vi "EHL Undo Filter - Value Change MHLC.vi"(8 "error in (no error)":errorcluster, 11 "Message Log in":refnum<class "Message Log.lvclass">) -> (0 "error out":errorcluster, 3 "Message Log out":refnum<class "Message Log.lvclass">)   [LabVIEW 2017, in "Message Log.lvclass"]
doc: "Remove last applied filter"
uses:
  Message Log.lvclass
  Message Log.lvclass/Message Log.ctl
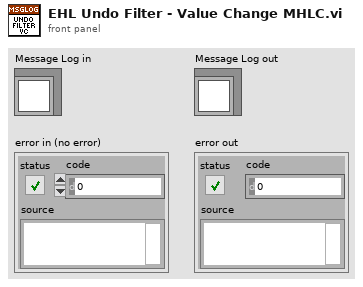
[diagram p1: front panel]
types:
  T1 = typedef "Message Log.lvclass/Message Log Filter Data.ctl" = cluster{"Element":string, "Column":T2, "Filter Type":T3}
  T2 = typedef "Message Log.lvclass/Message Log Columns.ctl" = enum16{"Count (sec)", "Time/Date", "Enque Worker", "Enque Case", "Deque Worker", "Deque Case", "Priority", "Message"}
  T3 = typedef "Message Log.lvclass/String Filter Type.ctl" = enum16{"string only", "match pattern"}
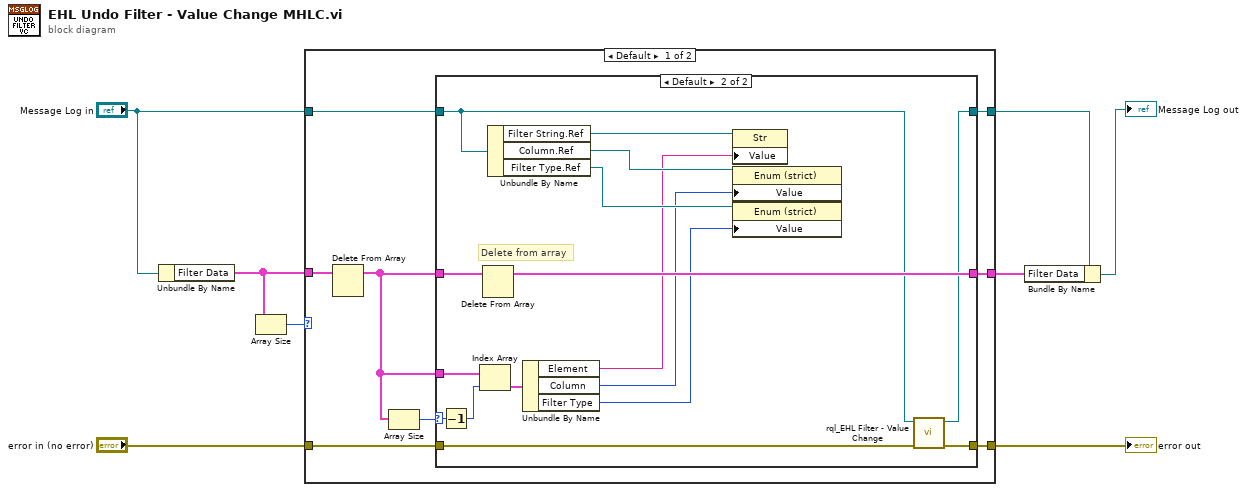
[diagram p0: block diagram]
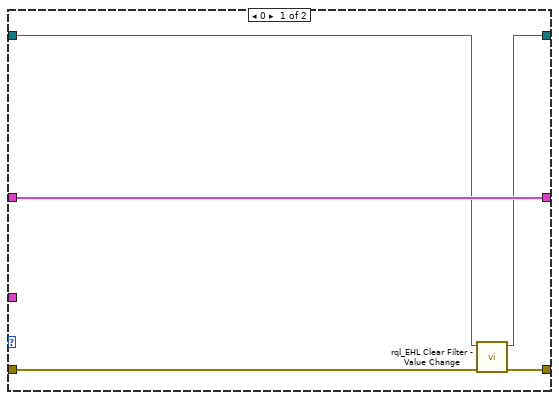
[diagram p2: hidden frame]
diagram:
  n1 = Unbundle By Name("Message Log in") -> ("Filter Data"=w2:T1[])
  n2 = Array Size(array=w2) -> (size(s)=w1:i32)
  n3 = case shown="Default" w1 {
    tunnel: w2 -> [w16 w40]
    tunnel: [w14 w40] -> w3
    tunnel: [w12 w39] -> w7
    tunnel: "error in (no error)" -> [w11 w39]
    tunnel: [w10 w38] -> w4
    tunnel: "Message Log in" -> [w9 w38]
    frame Default {
      n4 = Delete From Array(array=w16) -> (array with subset deleted=w13:T1[])  [unwired: 2 in, 1 out]
      n5 = Array Size(array=w13) -> (size(s)=w15:i32)
      n6 = case shown="Default" w15 {
        selector: w15 -> [_ w35]
        tunnel: w13 -> [_ w36]
        tunnel: [w21 w33] -> w14
        tunnel: w13 -> [w21 w32]
        tunnel: [w19 w31] -> w12
        tunnel: w11 -> [w20 w30]
        tunnel: [w17 w29] -> w10
        tunnel: w9 -> [w18 w28]
        frame 0 {
          n7 = call "rql_EHL Clear Filter - Value Change.vi"("error in"=w20, "Message Log in"=w18) -> ("error out"=w19:errorcluster, "dup Message Log out"=w17:refnum<class "Message Log.lvclass">)  [unwired: 8 in]
        }
        frame Default {
          # "Delete from array"
          n8 = Decrement(x=w35) -> (x-1=w34:i32)
          n9 = Index Array(array=w36, index=w34) -> (element=w37:T1)
          n10 = Delete From Array(array=w32) -> (array with subset deleted=w33:T1[])  [unwired: 2 in, 1 out]
          n11 = Unbundle By Name(w28) -> ("Filter String.Ref"=w27:refnum<vi>, "Column.Ref"=w26:refnum<vi>, "Filter Type.Ref"=w25:refnum<vi>)
          n12 = Unbundle By Name(w37) -> ("Element"=w24:string, "Column"=w23:T2, "Filter Type"=w22:T3)
          n13 = property class="Str"(reference=w27, "Value"=w24) -> ()  [unwired: 1 in, 2 out]
          n14 = property class="Enum (strict)"(reference=w26, "Value"=w23) -> ()  [unwired: 1 in, 2 out]
          n15 = property class="Enum (strict)"(reference=w25, "Value"=w22) -> ()  [unwired: 1 in, 2 out]
          n16 = call "rql_EHL Filter - Value Change.vi"("error in"=w30, "Message Log in"=w28) -> ("error out"=w31:errorcluster, "dup Message Log out"=w29:refnum<class "Message Log.lvclass">)  [unwired: 8 in]
        }
      }
    }
    frame 0 {
      # "array empty. do nothing"
    }
  }
  "error out" <- w7
  n17 = Bundle By Name(cluster=w4, "Filter Data"=w3) -> (→"Message Log out":refnum<class "Message Log.lvclass">)
